vi "AppendWaveformWrite.vi"(10 "WFM in in":T1, 11 "index of element":i32) -> (3 "WFM out":T1)   [LabVIEW 2016]
uses:
  SMOs/DAQ/Typedefs/PublicEvents--DAQ.Write.ctl
  SMOs/DAQ/DAQ.lvclass
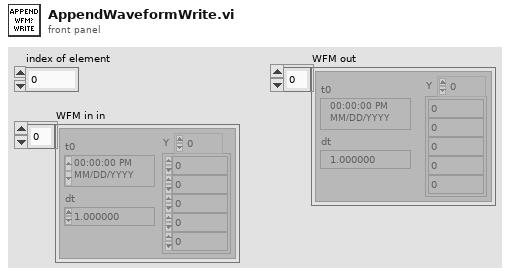
[diagram p1: front panel]
types:
  T1 = typedef "DAQ.lvclass/PublicEvents--DAQ.Write.ctl" = waveform(dbl)[]
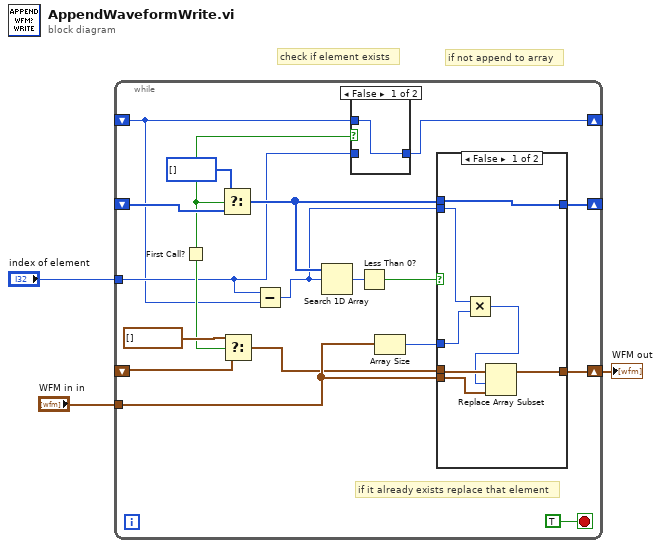
[diagram p0: block diagram]
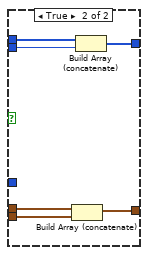
[diagram p3: hidden frame]
diagram:
  # "if not append to array"
  # "check if element exists"
  n1 = while {
    tunnel: "WFM in in" -> [w16]
    tunnel: "index of element" -> [w6]
    shift-right: [w20] -> _
    shift-left: _ -> [w14]
    shift-right: [w18] -> w3
    shift-left: _ -> [w12]
    shift-right: [w7] -> _
    shift-left: _ -> [w5]
    stop <- TRUE stop-if-true
    # "if it already exists replace that element"
    n2 = First Call?() -> (First Call?: T/F=w8:bool)
    n3 = Select(t=i32[] [], s=w8, f=w14) -> (s? t:f=w9:i32[])
    n4 = Select(t=T1 [] ("WFM in"), s=w8, f=w12) -> (s? t:f=w11:T1)
    n5 = Subtract(x=w6, y=w5) -> (x-y=w4:i32)
    n6 = Search 1D Array(1D array=w9, element=w4) -> (index of element=w19:i32)  [unwired: 1 in]
    n7 = case shown="False" w8 {
      tunnel: [w22 w23] -> w7
      tunnel: w6 -> [_ w23]
      tunnel: w5 -> [w22 _]
      frame False {
      }
      frame True {
      }
    }
    n8 = Less Than 0?(x=w19) -> (x < 0?=w17:bool)
    n9 = Array Size(array=w16) -> (size(s)=w15:i32)
    n10 = case shown="False" w17 {
      tunnel: [w24 w36] -> w20
      tunnel: w4 -> [w27 w35]
      tunnel: w9 -> [w24 w34]
      tunnel: w16 -> [w29 w33]
      tunnel: [w28 w32] -> w18
      tunnel: w11 -> [w30 w31]
      tunnel: w15 -> [w26 _]
      frame False {
        n11 = Multiply(x=w27, y=w26) -> (x*y=w25:i32)
        n12 = Replace Array Subset(array=w30, new element=w29, index=w25) -> (w28:T1)
      }
      frame True {
        n13 = Build Array (concatenate)(w31, w33) -> (w32:T1)
        n14 = Build Array (concatenate)(w34, w35) -> (w36:i32[])
      }
    }
  }
  "WFM out" <- w3
